vi "DEMO.vi"() -> ()   [LabVIEW 2018, in "VXMMotionManager.lvclass"]
uses:
  VXMMotionManager.lvclass
  VSMx2/VXMx2.lvclass
  <instrlib>/Velmex VXM/Public/VXM Axis.ctl
  <instrlib>/Velmex VXM/Velmex VXM.lvlib
  VXMCfg/sub-syst.n.ctl
  sub-systems/sub-systems.lvclass
  Position.ctl
panel:
  out "Axis Number":i32
  out "error out":errorcluster
  out "i":i32=63
  in  "stop":bool
  in  "Positions, steps":T1={"X, mm"=5000.0, "Y, mm"=6000.0, "Z, mm"=7000.0, "T, deg"=8000.0}
  in  "Position Array":T2(array[cluster])
  in  "HomeOffset":T3
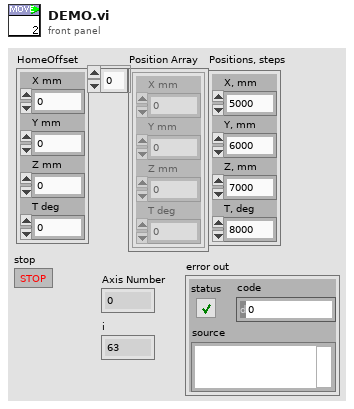
[diagram p1: front panel]
types:
  T1 = typedef "Position.ctl" = cluster{"X, mm":dbl, "Y, mm":dbl, "Z, mm":dbl, "T, deg":dbl}
  T2 = cluster{"X mm":dbl, "Y mm":dbl, "Z mm":dbl, "T deg":dbl}[]
  T3 = cluster{"X mm":dbl, "Y mm":dbl, "Z mm":dbl, "T deg":dbl}
  T4 = typedef "sub-syst.n.ctl" = cluster{"Addr":string, "Enable":bool, "X scale eng./step":dbl, "Y scale eng./step":dbl, "Z scale eng./step":dbl, "T scale eng./step":dbl, "X units":string, "Y units":string, "Z units":string, "T units":string, "X Jog":dbl, "Y Jog":dbl, "Z Jog":dbl, "T Jog":dbl, "X-1 Name":string, "Y-2 Name":string, "Z-3 Name":string, "T-4 Name":string, "VXM (1-4)":i32}
  T5 = typedef "Velmex VXM.lvlib/VXM Axis.ctl" = u16
  T6 = cluster{"X mm/step":dbl, "Y mm/step":dbl, "Z mm/step":dbl, "T deg/step":dbl}
  T7 = cluster{"X step":dbl, "Y step":dbl, "Z step":dbl, "T step":dbl}
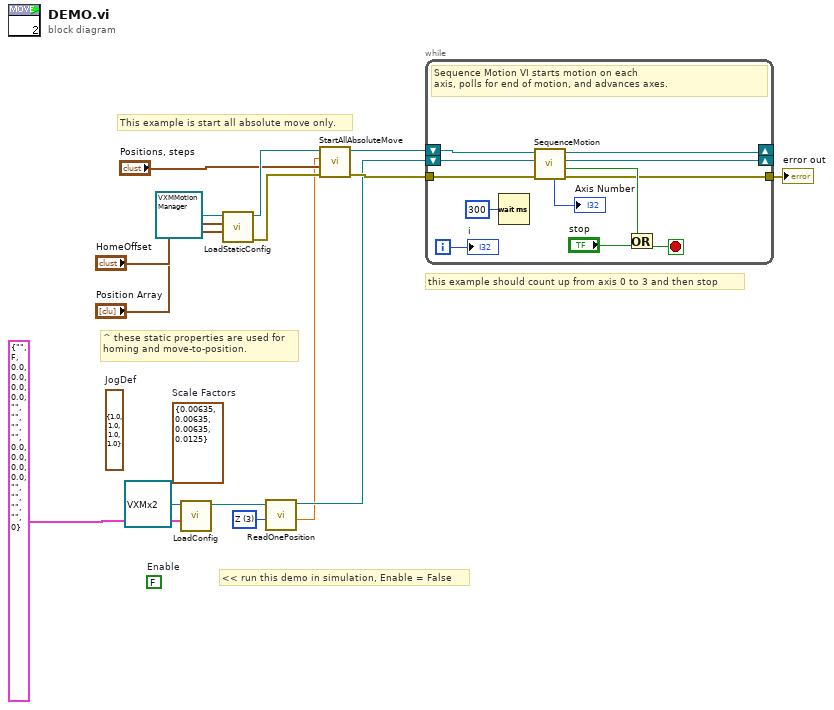
[diagram p0: block diagram]
diagram:
  w5 = T5 3 items=["X"=1, "Y"=2, "Z"=3, "Rotary"=4] ("Axis (1..4)")
  (unwired) T6 {"X mm/step"=0.00635, "Y mm/step"=0.00635, "Z mm/step"=0.00635, "T deg/step"=0.0125}  # Scale Factors
  (unwired) T7 {"X step"=1.0, "Y step"=1.0, "Z step"=1.0, "T step"=1.0}  # JogDef
  (unwired) FALSE  # Enable
  # "this example should count up from axis 0 to 3 and then stop"
  # "<< run this demo in simulation, Enable = False"
  # "This example is start all absolute move only."
  # "^ these static properties are used for \nhoming and move-to-position."
  n1 = call "LoadConfig.vi"("sub-syst Cfg"=T4 {"Addr"="", "Enable"=FALSE, "X scale eng./step"=0.0, "Y scale eng./step"=0.0, "Z scale eng./step"=0.0, "T scale eng./step"=0.0, "X units"="", "Y units"="", "Z units"="", "T units"="", "X Jog"=0.0, "Y Jog"=0.0, "Z Jog"=0.0, "T Jog"=0.0, "X-1 Name"="", "Y-2 Name"="", "Z-3 Name"="", "T-4 Name"="", "VXM (1-4)"=0}, "VXMx2 in"=refnum<class "VXMx2.lvclass"> refnum) -> ("VXMx2 out"=w4:refnum<class "VXMx2.lvclass">)  [unwired: 8 in, 1 out]
  n2 = call "LoadStaticConfig.vi"(9:"Position Array", 10:"HomeOffset", "VXMMotionManager in"=refnum<class "VXMMotionManager.lvclass"> refnum) -> ("error out"=w10:errorcluster, "VXMMotionManager out"=w12:refnum<class "VXMMotionManager.lvclass">)  [unwired: 7 in]
  n3 = call "ReadOnePosition.vi"("Axis (1..4)"=w5, "VXMx2 in"=w4) -> ("Position, eng units"=w2:dbl, "VXMx2 out"=w3:refnum<class "VXMx2.lvclass">)  [unwired: 7 in, 1 out]
  n4 = call "StartAllAbsoluteMove.vi"("error in (no error)"=w10, "Positions, steps"="Positions, steps", "Current Z pos., mm"=w2, "VXMMotionManager in"=w12) -> ("error out"=w8:errorcluster, "VXMMotionManager out"=w7:refnum<class "VXMMotionManager.lvclass">)  [unwired: 6 in]
  n5 = while {
    tunnel: w8 -> [w27]
    shift-right: [w20] -> _
    shift-left: w3 -> [w21]
    shift-right: [w18] -> _
    shift-left: w7 -> [w19]
    tunnel: [w17] -> w6
    i -> [w22]
    stop <- w24 stop-if-true
    # "Sequence Motion VI starts motion on each\naxis, polls for end of motion, and advances axes."
    n6 = Wait (ms)(milliseconds to wait=u32 300) -> ()  [unwired: 1 out]
    n7 = call "SequenceMotion.vi"("error in (no error)"=w27, "sub-systems in"=w21, "VXMMotionManager in"=w19) -> ("error out"=w17:errorcluster, "Motions Finished = T"=w23:bool, "sub-systems out"=w20:refnum<class "sub-systems.lvclass">, "VXMMotionManager out"=w18:refnum<class "VXMMotionManager.lvclass">, "Axis Number"=→"Axis Number":i32)  [unwired: 3 in, 1 out]
    n8 = Or(x=w23, y="stop") -> (x .or. y?=w24:bool)
    "i" <- w22
  }
  "error out" <- w6
